vi "Server.vi"() -> ()   [LabVIEW 2021]
uses:
  <vilib>/Utility/miscctls.llb/LVPositionTypeDef.ctl
  MessageType.ctl
  <vilib>/event_ctls.llb/eventsource.ctl
panel:
  in  "stop":bool
  in  "State Change":bool=TRUE
  out "GS":enum16{"Player 1 shoot", "Player 2 Shoot"}(ring)
  out "Status":string
  out "Player 1":u8
  out "Player 2 Score":u8
  in  "Goal Post":cluster{"left":i16, "Size":i16}={"left"=110, "Size"=125}
  out "Goal Post":T1={"left"=110, "top"=0, "right"=235, "bottom"=15}
  out "Box":T1={"left"=139, "top"=147, "right"=181, "bottom"=180}
  out "goal?":bool=TRUE
  out "Del GK":dbl
  out "Defend":bool
  in  "GK":cluster{"horizontal":dbl, "vertical":dbl}={"horizontal"=175.0, "vertical"=20.0}
  in  "Box Size":cluster{"horizontal":dbl, "Vertical":dbl}={"horizontal"=21.0, "Vertical"=33.0}
  in  "Reset":bool
  out "del x":dbl=-0.26666666666666666
  in  "wait":u32=10
  in  "shot?":bool
  in  "Power":dbl(slide)=1.4141414141414141 scale=0.0..10.0
  in  "Ball Size":i16=9
  in  "Ball":cluster{"horizontal":dbl, "vertical":dbl}={"horizontal"=160.0, "vertical"=180.0}
  in  "Shoot":bool
  out "Ground":picture
  # "PLAYER 1"
  # "Misc. Controls"
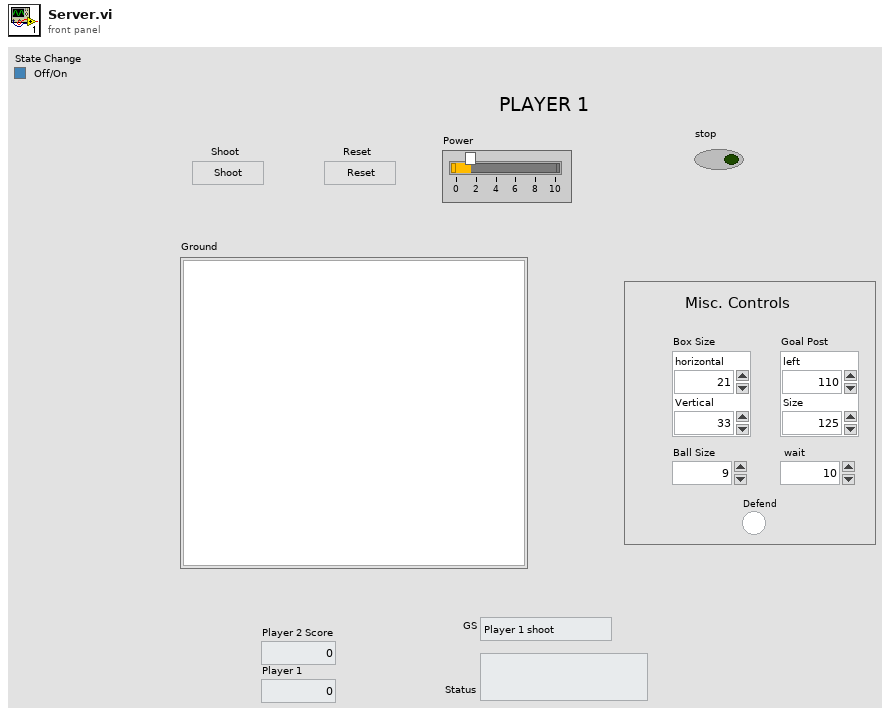
[diagram p1: front panel]
types:
  T1 = cluster{"left":i16, "top":i16, "right":i16, "bottom":i16}
  T2 = typedef "MessageType.ctl" = enum16{"Shoot", "Defend", "Reset", "Score"}
  T3 = typedef "LVPositionTypeDef.ctl" = cluster{"Left":i32, "Top":i32}
  T4 = typedef "LVPoint32TypeDef.ctl" = cluster{"Horizontal":i32, "Vertical":i32}
  T5 = typedef "eventsource.ctl" = u32
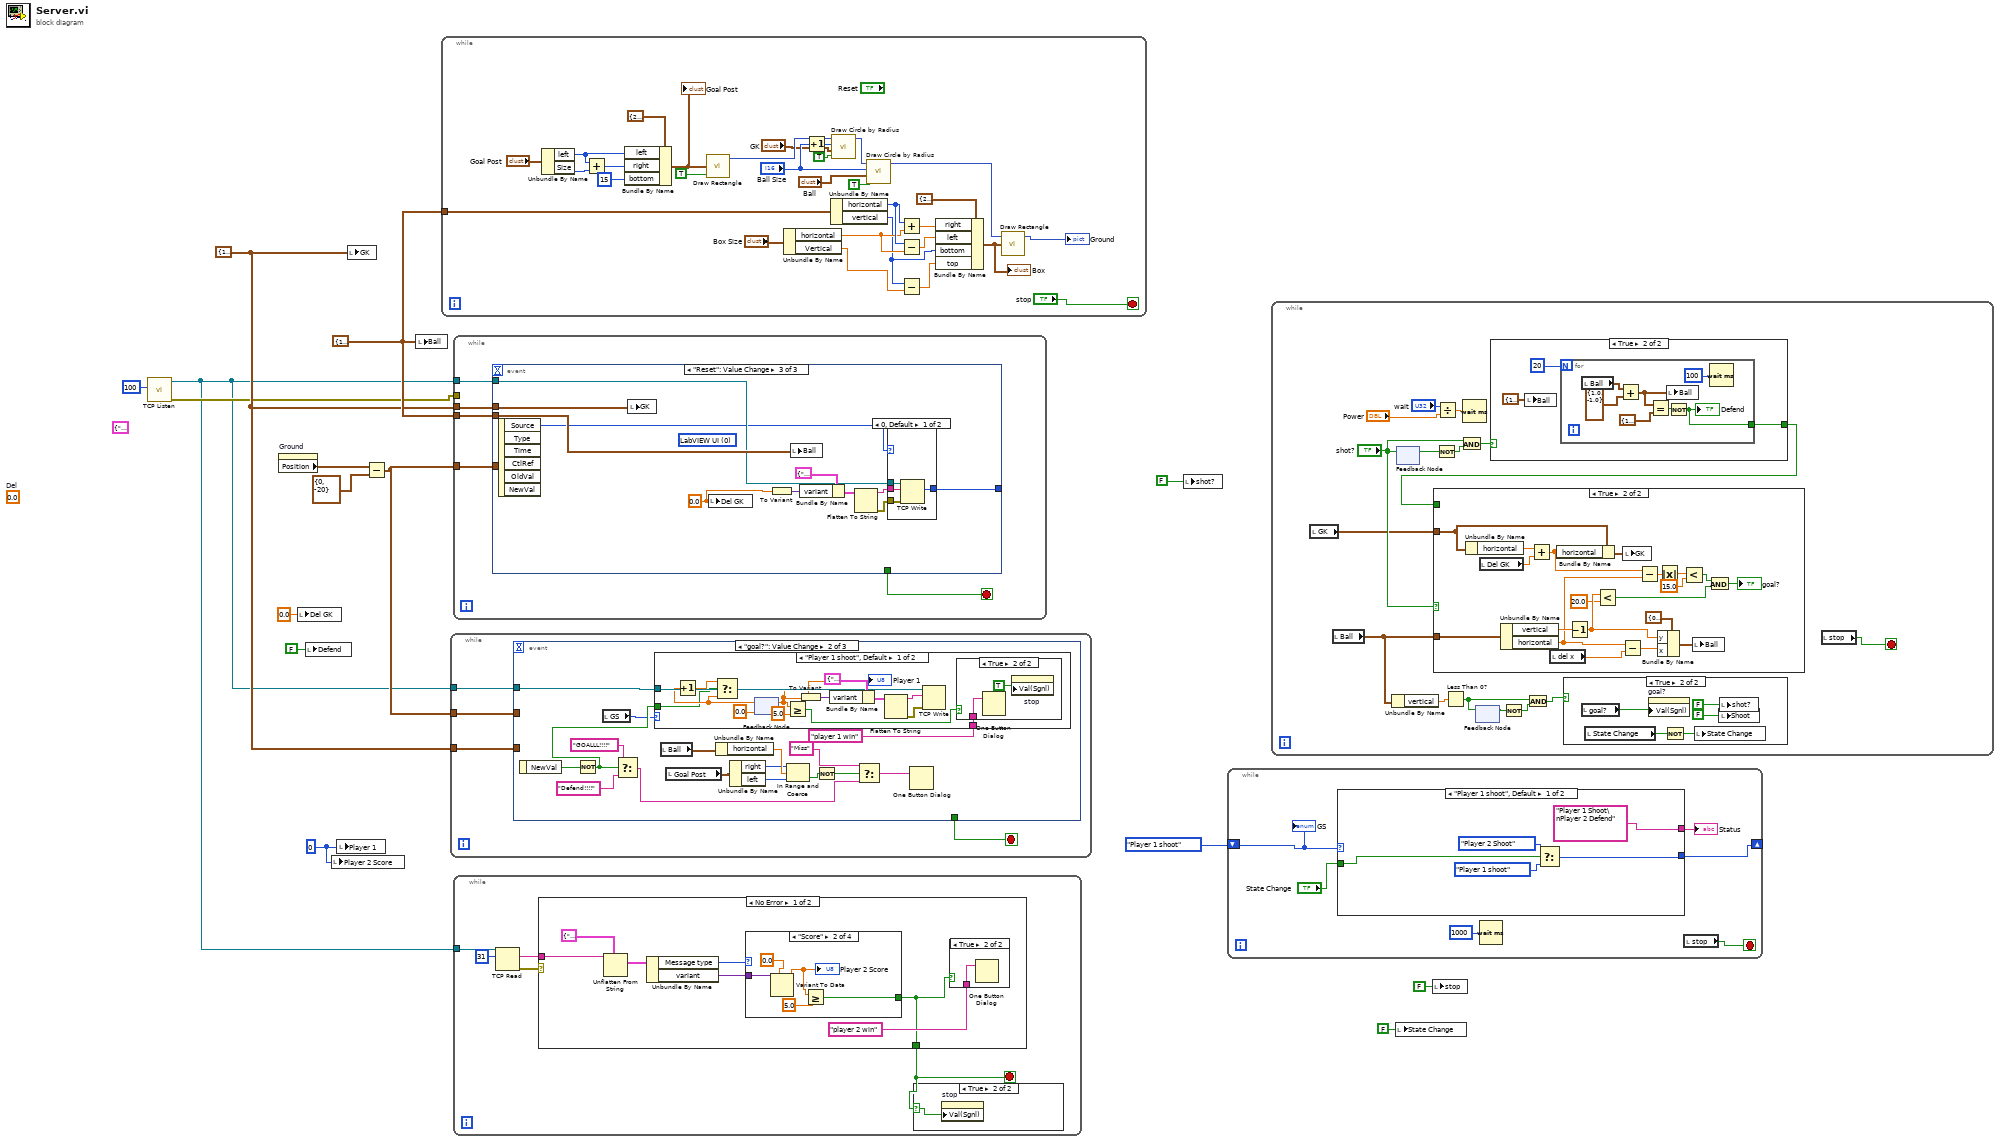
[diagram p0: block diagram]
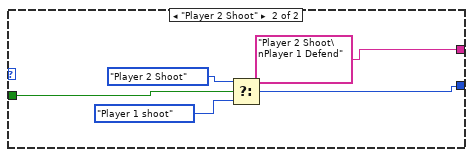
[diagram p2: hidden frame]
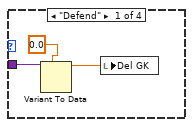
[diagram p5: hidden frame]
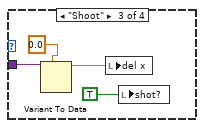
[diagram p6: hidden frame]
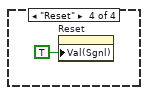
[diagram p7: hidden frame]
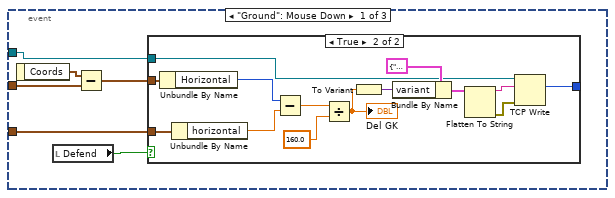
[diagram p9: hidden frame]
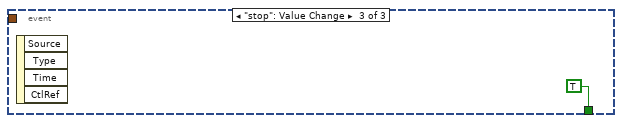
[diagram p13: hidden frame]
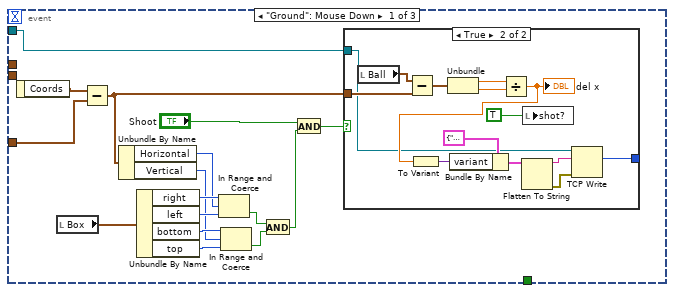
[diagram p17: hidden frame]
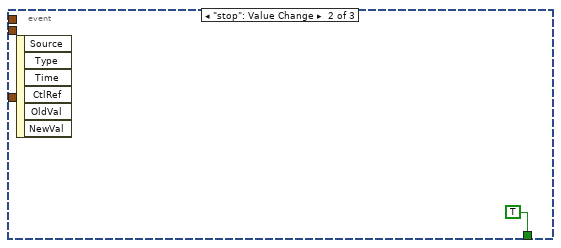
[diagram p19: hidden frame]
diagram:
  w4 = u8 0 ("Player 1")
  (unwired) 0.0  # Del
  (unwired) cluster{"Message type":T2, "variant":variant} {"Message type"=enum."Reset", "variant"=variant}
  w9 = cluster{"horizontal":dbl, "vertical":dbl} {"horizontal"=175.0, "vertical"=20.0} ("GK")
  w12 = cluster{"horizontal":i16, "vertical":i16} {"horizontal"=160, "vertical"=180} ("Ball")
  n1 = call <vilib>:"TCP Listen.vi"("port"=u16 100) -> ("error out"=w6:errorcluster, "connection ID"=w5:refnum<k5>)  [unwired: 6 in, 3 out]
  n2 = property on="Ground" class="Pict"() -> ("Position"=w14:T3)  [unwired: 2 in, 2 out]
  n3 = local write "Del GK"(0.0 ("Del GK")) -> ()
  n4 = local write "Defend"(FALSE ("def")) -> ()
  n5 = local write "Player 2 Score"(w4) -> ()
  n6 = local write "Player 1"(w4) -> ()
  n7 = local write "GK"(w9) -> ()
  n8 = Subtract(x=w14, y=T3 {"Left"=0, "Top"=-20}) -> (x-y=w11:T3)
  n9 = local write "Ball"(w12) -> ()
  n10 = while {
    tunnel: w12 -> [w26]
    stop <- "stop" stop-if-true
    n11 = Unbundle By Name("Goal Post") -> ("left"=w18:i16, "Size"=w17:i16)
    n12 = Add(x=w18, y=w17) -> (x+y=w41:i16)
    n13 = Bundle By Name(cluster=T1 {"left"=22, "top"=0, "right"=10, "bottom"=10} ("rect"), "left"=w18, "right"=w41, "bottom"=i16 15) -> (w42:T1)
    "Goal Post" <- w42
    n14 = call <vilib>:"Draw Rectangle.vi"("rect"=w42, "fill?(F)"=TRUE) -> ("new picture"=w23:picture)  [unwired: 7 in]
    n15 = Unbundle By Name("Box Size") -> ("horizontal"=w34:dbl, "Vertical"=w31:dbl)
    n16 = Increment(x="Ball Size") -> (x+1=w20:i16)
    n17 = Unbundle By Name(w26) -> ("horizontal"=w35:i16, "vertical"=w33:i16)
    n18 = call <vilib>:"Draw Circle by Radius.vi"("fill?(F)"=TRUE, "pixel center"="GK", "radius"=w20, "picture"=w23) -> ("new picture"=w21:picture)  [unwired: 7 in]
    n19 = call <vilib>:"Draw Circle by Radius.vi"("fill?(F)"=TRUE, "pixel center"="Ball", "radius"="Ball Size", "picture"=w21) -> ("new picture"=w28:picture)  [unwired: 7 in]
    n20 = Add(x=w35, y=w34) -> (x+y=w36:dbl)
    n21 = Subtract(x=w35, y=w34) -> (x-y=w32:dbl)
    n22 = Subtract(x=w33, y=w31) -> (x-y=w30:dbl)
    n23 = Bundle By Name(cluster=T1 {"left"=22, "top"=0, "right"=10, "bottom"=10} ("rect"), "right"=w36, "left"=w32, "bottom"=w33, "top"=w30) -> (w29:T1)
    "Box" <- w29
    n24 = call <vilib>:"Draw Rectangle.vi"("picture"=w28, "rect"=w29) -> ("new picture"=→"Ground":picture)  [unwired: 7 in]
  }
  n25 = while {
    tunnel: w11 -> [w49]
    tunnel: w9 -> [w48]
    tunnel: w5 -> [w47]
    stop <- w46 stop-if-true
    n26 = event shown="[1] \"goal?\": Value Change" {
      selector: _ -> [_ _ _]
      dyn-events: _ -> [_ _ _]
      timeout: _ -> [_ _ _]
      tunnel: w49 -> [w54 _ _]
      tunnel: w48 -> [w52 _ _]
      tunnel: w47 -> [w50 w73 _]
      tunnel: [_ _ TRUE] -> w46
      event "Ground": Mouse Down {
        n27 = event-data() -> ("Coords"=w55:T4)  [unwired: 1 in]
        n28 = local read "Defend"() -> (w51:bool)
        n29 = Subtract(x=w55, y=w54) -> (x-y=w53:T4)
        n30 = case shown="True" w51 {
          tunnel: w53 -> [_ w69]
          tunnel: w52 -> [_ w68]
          tunnel: w50 -> [_ w58]
          tunnel: [_ w56] -> _
          frame False {
          }
          frame True {
            n31 = Unbundle By Name(w69) -> ("Horizontal"=w67:i32)
            n32 = Unbundle By Name(w68) -> ("horizontal"=w66:dbl)
            n33 = Subtract(x=w67, y=w66) -> (x-y=w65:dbl)
            n34 = Divide(x=w65, y=160.0) -> (x/y=w57:dbl)
            "Del GK" <- w57
            n35 = To Variant(anything=w57) -> (Variant=w62:variant)
            n36 = Bundle By Name(cluster=cluster{"Message type":T2, "variant":variant} {"Message type"=enum."Defend", "variant"=variant}, "variant"=w62) -> (w61:cluster{"Message type":T2, "variant":variant})
            n37 = Flatten To String(anything=w61) -> (data string=w59:string, error out=w60:errorcluster)  [unwired: 3 in, 1 out]
            n38 = TCP Write(connection ID=w58, data in=w59, error in (no error)=w60) -> (bytes written=w56:i32)  [unwired: 1 in, 2 out]
          }
        }
      }
      event "goal?": Value Change {
        n39 = event-data() -> ("NewVal"=w86:bool)  [unwired: 1 in]
        n40 = Not(x=w86) -> (.not. x?=w72:bool)
        n41 = local read "GS"() -> (w71:enum16{"Player 1 shoot", "Player 2 Shoot"})
        n42 = Select(t="GOALLL!!!!", s=w72, f="Defend!!!!") -> (s? t:f=w75:string)
        n43 = case shown="\"Player 1 shoot\", Default" w71 {
          tunnel: w73 -> [w95 _]
          tunnel: w72 -> [w92 _]
          tunnel: "player 1 win" -> [w87 _]
          frame "Player 1 shoot", Default {
            n44 = feedback #1(0.0) -> (w93:dbl)
            n45 = Increment(x=w93) -> (x+1=w94:dbl)
            n46 = Select(t=w94, s=w92, f=w93) -> (s? t:f=w90:dbl)
            "Player 1" <- w90
            n47 = feedback-in #1(w90) -> ()
            n48 = Greater Or Equal?(x=w90, y=5.0) -> (x >= y?=w88:bool)
            n49 = To Variant(anything=w90) -> (Variant=w99:variant)
            n50 = Bundle By Name(cluster=cluster{"Message type":T2, "variant":variant} {"Message type"=enum."Score", "variant"=variant}, "variant"=w99) -> (w98:cluster{"Message type":T2, "variant":variant})
            n51 = Flatten To String(anything=w98) -> (data string=w96:string, error out=w97:errorcluster)  [unwired: 3 in, 1 out]
            n52 = TCP Write(connection ID=w95, data in=w96, error in (no error)=w97) -> ()  [unwired: 1 in, 3 out]
            n53 = case shown="True" w88 {
              tunnel: w87 -> [_ w102]
              frame False {
              }
              frame True {
                n54 = One Button Dialog(message=w102) -> ()  [unwired: 1 in, 1 out]
                n55 = property on="stop" class="Bool (strict)"("Val(Sgnl)"=TRUE ("Value (Signaling)")) -> ()  [unwired: 2 in, 2 out]
              }
            }
          }
          frame "Player 2 Shoot" {
          }
        }
        n56 = local read "Ball"() -> (w79:cluster{"horizontal":dbl, "vertical":dbl})
        n57 = local read "Goal Post"() -> (w80:T1)
        n58 = Unbundle By Name(w79) -> ("horizontal"=w83:dbl)
        n59 = Unbundle By Name(w80) -> ("right"=w81:i16, "left"=w82:i16)
        n60 = In Range and Coerce(upper limit=w81, x=w83, lower limit=w82) -> (In Range?=w78:bool)  [unwired: 1 out]
        n61 = Not(x=w78) -> (.not. x?=w74:bool)
        n62 = Select(t="Miss", s=w74, f=w75) -> (s? t:f=w76:string)
        n63 = One Button Dialog(message=w76) -> ()  [unwired: 1 in, 1 out]
      }
      event "stop": Value Change {
        n64 = event-data() -> ()  [unwired: 1 in, 4 out]
      }
    }
  }
  n65 = while {
    tunnel: w11 -> [w108]
    tunnel: w12 -> [w107]
    tunnel: w9 -> [w106]
    tunnel: w5 -> [w105]
    tunnel: w6 -> [_]
    stop <- w104 stop-if-true
    n66 = event shown="[2] \"Reset\": Value Change" {
      selector: _ -> [_ _ _]
      dyn-events: _ -> [_ _ _]
      timeout: _ -> [_ _ _]
      tunnel: w108 -> [w122 _ _]
      tunnel: w107 -> [_ _ w150]
      tunnel: w106 -> [_ _ w149]
      tunnel: w105 -> [w110 _ w143]
      tunnel: [_ _ w141] -> _
      tunnel: [_ TRUE _] -> w104
      event "Ground": Mouse Down {
        n67 = event-data() -> ("Coords"=w123:T4)  [unwired: 1 in]
        n68 = local read "Box"() -> (w121:T1)
        n69 = Subtract(x=w123, y=w122) -> (x-y=w116:T4)
        n70 = Unbundle By Name(w116) -> ("Horizontal"=w115:i32, "Vertical"=w114:i32)
        n71 = Unbundle By Name(w121) -> ("right"=w120:i16, "left"=w119:i16, "bottom"=w118:i16, "top"=w117:i16)
        n72 = In Range and Coerce(upper limit=w120, x=w115, lower limit=w119) -> (In Range?=w112:bool)  [unwired: 1 out]
        n73 = In Range and Coerce(upper limit=w118, x=w114, lower limit=w117) -> (In Range?=w113:bool)  [unwired: 1 out]
        n74 = And(x=w112, y=w113) -> (x .and. y?=w109:bool)
        n75 = And(x="Shoot", y=w109) -> (x .and. y?=w111:bool)
        n76 = case shown="True" w111 {
          tunnel: w116 -> [_ w137]
          tunnel: w110 -> [_ w126]
          tunnel: [_ w125] -> _
          frame False {
          }
          frame True {
            n77 = local read "Ball"() -> (w136:cluster{"horizontal":dbl, "vertical":dbl})
            n78 = Subtract(x=w136, y=w137) -> (x-y=w135:cluster{dbl, dbl})
            n79 = Unbundle(w135) -> (w134:dbl, w133:dbl)
            n80 = Divide(x=w134, y=w133) -> (x/y=w131:dbl)
            "del x" <- w131
            n81 = To Variant(anything=w131) -> (Variant=w130:variant)
            n82 = Bundle By Name(cluster=cluster{"Message type":T2, "variant":variant} {"Message type"=enum."Shoot", "variant"=variant}, "variant"=w130) -> (w129:cluster{"Message type":T2, "variant":variant})
            n83 = Flatten To String(anything=w129) -> (data string=w127:string, error out=w128:errorcluster)  [unwired: 3 in, 1 out]
            n84 = local write "shot?"(TRUE ("Checkbox")) -> ()
            n85 = TCP Write(connection ID=w126, data in=w127, error in (no error)=w128) -> (bytes written=w125:i32)  [unwired: 1 in, 2 out]
          }
        }
      }
      event "stop": Value Change {
        n86 = event-data() -> ()  [unwired: 1 in, 6 out]
      }
      event "Reset": Value Change {
        (unwired) T5 0 items=["LabVIEW UI"=0, "ActiveX"=1, "User Event"=25] ("Source")
        w142 = 0.0
        n87 = event-data() -> ("Source"=w140:T5)  [unwired: 1 in, 5 out]
        n88 = local write "GK"(w149) -> ()
        n89 = local write "Del GK"(w142) -> ()
        n90 = To Variant(anything=w142) -> (Variant=w147:variant)
        n91 = local write "Ball"(w150) -> ()
        n92 = Bundle By Name(cluster=cluster{"Message type":T2, "variant":variant} {"Message type"=enum."Reset", "variant"=variant}, "variant"=w147) -> (w146:cluster{"Message type":T2, "variant":variant})
        n93 = Flatten To String(anything=w146) -> (data string=w144:string, error out=w145:errorcluster)  [unwired: 3 in, 1 out]
        n94 = case shown="0, Default" w140 {
          tunnel: w145 -> [w154 _]
          tunnel: w144 -> [w153 _]
          tunnel: w143 -> [w152 _]
          tunnel: [w151 _] -> w141
          frame 0, Default {
            n95 = TCP Write(connection ID=w152, data in=w153, error in (no error)=w154) -> (bytes written=w151:i32)  [unwired: 1 in, 2 out]
          }
          frame 1 {
          }
        }
      }
    }
  }
  n96 = while {
    tunnel: w5 -> [w159]
    stop <- w155 stop-if-true
    n97 = TCP Read(connection ID=w159, bytes to read=31) -> (data out=w156:string, error out=w157:errorcluster)  [unwired: 3 in, 1 out]
    n98 = case shown="No Error" w157 {
      tunnel: w156 -> [w167 _]
      tunnel: [w161 _] -> w155
      frame No Error {
        n99 = Unflatten From String(type=cluster{"Message type":T2, "variant":variant} {"Message type"=enum."Defend", "variant"=variant}, binary string=w167) -> (value=w165:cluster{"Message type":T2, "variant":variant})  [unwired: 3 in, 2 out]
        n100 = Unbundle By Name(w165) -> ("Message type"=w164:T2, "variant"=w163:variant)
        n101 = case shown="\"Score\"" w164 {
          tunnel: w163 -> [w171 w176 w180 _]
          tunnel: [_ w172 _ _] -> w161
          frame "Defend" {
            n102 = Variant To Data(type=0.0 ("x/y"), Variant=w171) -> (data=w169:dbl)  [unwired: 1 in, 1 out]
            n103 = local write "Del GK"(w169) -> ()
          }
          frame "Score" {
            n104 = Variant To Data(type=0.0 ("x/y"), Variant=w176) -> (data=w174:dbl)  [unwired: 1 in, 1 out]
            "Player 2 Score" <- w174
            n105 = Greater Or Equal?(x=w174, y=5.0) -> (x >= y?=w172:bool)
          }
          frame "Shoot" {
            n106 = Variant To Data(type=0.0 ("x/y"), Variant=w180) -> (data=w178:dbl)  [unwired: 1 in, 1 out]
            n107 = local write "del x"(w178) -> ()
            n108 = local write "shot?"(TRUE ("Checkbox")) -> ()
          }
          frame "Reset" {
            n109 = property on="Reset" class="Bool (strict)"("Val(Sgnl)"=TRUE ("Value (Signaling)")) -> ()  [unwired: 2 in, 2 out]
          }
        }
        n110 = case shown="True" w161 {
          tunnel: "player 2 win" -> [_ w168]
          frame False {
          }
          frame True {
            n111 = One Button Dialog(message=w168) -> ()  [unwired: 1 in, 1 out]
          }
        }
      }
      frame Error {
      }
    }
    n112 = case shown="True" w155 {
      selector: w155 -> [_ w160]
      frame False {
      }
      frame True {
        n113 = property on="stop" class="Bool (strict)"("Val(Sgnl)"=w160) -> ()  [unwired: 2 in, 2 out]
      }
    }
  }
  n114 = local write "shot?"(FALSE ("Checkbox")) -> ()
  n115 = while {
    shift-right: [w184] -> _
    shift-left: enum16{"Player 1 shoot", "Player 2 Shoot"}."Player 1 shoot" -> [w187]
    stop <- w182 stop-if-true
    n116 = case shown="\"Player 1 shoot\", Default" w187 {
      tunnel: ["Player 1 Shoot\nPlayer 2 Defend" "Player 2 Shoot\nPlayer 1 Defend"] -> w186
      tunnel: [w189 w194] -> w184
      tunnel: "State Change" -> [w188 w193]
      frame "Player 1 shoot", Default {
        n117 = Select(t=enum16{"Player 1 shoot", "Player 2 Shoot"}."Player 2 Shoot", s=w188, f=enum16{"Player 1 shoot", "Player 2 Shoot"}."Player 1 shoot") -> (s? t:f=w189:enum16{"Player 1 shoot", "Player 2 Shoot"})
      }
      frame "Player 2 Shoot" {
        n118 = Select(t=enum16{"Player 1 shoot", "Player 2 Shoot"}."Player 2 Shoot", s=w193, f=enum16{"Player 1 shoot", "Player 2 Shoot"}."Player 1 shoot") -> (s? t:f=w194:enum16{"Player 1 shoot", "Player 2 Shoot"})
      }
    }
    "Status" <- w186
    n119 = Wait (ms)(milliseconds to wait=u32 1000) -> ()  [unwired: 1 out]
    n120 = local read "stop"() -> (w182:bool)
    "GS" <- w187
  }
  n121 = while {
    stop <- w198 stop-if-true
    n122 = local read "GK"() -> (w204:cluster{"horizontal":dbl, "vertical":dbl})
    n123 = local read "Ball"() -> (w210:cluster{"horizontal":dbl, "vertical":dbl})
    n124 = Unbundle By Name(w210) -> ("vertical"=w209:dbl)
    n125 = feedback-in #2("shot?") -> ()
    n126 = feedback #2() -> (w208:bool)  [unwired: 1 in]
    n127 = Not(x=w208) -> (.not. x?=w206:bool)
    n128 = Divide(x="wait", y="Power") -> (x/y=w212:dbl)
    n129 = Less Than 0?(x=w209) -> (x < 0?=w203:bool)
    n130 = And(x="shot?", y=w206) -> (x .and. y?=w205:bool)
    n131 = Wait (ms)(milliseconds to wait=w212) -> ()  [unwired: 1 out]
    n132 = feedback #3() -> (w201:bool)  [unwired: 1 in]
    n133 = feedback-in #3(w203) -> ()
    n134 = case shown="True" w205 {
      tunnel: [_ w214] -> w199
      frame False {
      }
      frame True {
        n135 = local write "Ball"(cluster{"horizontal":i16, "vertical":i16} {"horizontal"=140, "vertical"=200} ("Ball")) -> ()
        n136 = for {
          N: 20 -> [_]
          tunnel: [w217] -> w214
          n137 = local read "Ball"() -> (w223:cluster{"horizontal":dbl, "vertical":dbl})
          n138 = Add(x=w223, y=cluster{"horizontal":dbl, "vertical":dbl} {"horizontal"=1.0, "vertical"=-1.0}) -> (x+y=w220:cluster{"horizontal":dbl, "vertical":dbl})
          n139 = Equal?(x=w220, y=cluster{"horizontal":i16, "vertical":i16} {"horizontal"=160, "vertical"=180} ("Ball")) -> (x = y?=w219:bool)
          n140 = local write "Ball"(w220) -> ()
          n141 = Not(x=w219) -> (.not. x?=w217:bool)
          "Defend" <- w217
          n142 = Wait (ms)(milliseconds to wait=u32 100) -> ()  [unwired: 1 out]
        }
      }
    }
    n143 = case shown="True" "shot?" {
      tunnel: w210 -> [_ w243]
      tunnel: w204 -> [_ w242]
      tunnel: w199 -> [_ _]
      frame False {
      }
      frame True {
        n144 = Unbundle By Name(w242) -> ("horizontal"=w241:dbl)
        n145 = local read "Del GK"() -> (w240:dbl)
        n146 = Unbundle By Name(w243) -> ("vertical"=w247:dbl, "horizontal"=w235:dbl)
        n147 = Add(x=w241, y=w240) -> (x+y=w236:dbl)
        n148 = local read "del x"() -> (w248:dbl)
        n149 = Bundle By Name(cluster=w242, "horizontal"=w236) -> (w239:cluster{"horizontal":dbl, "vertical":dbl})
        n150 = Decrement(x=w247) -> (x-1=w238:dbl)
        n151 = Less?(x=w238, y=20.0) -> (x < y?=w230:bool)
        n152 = Subtract(x=w235, y=w248) -> (x-y=w245:dbl)
        n153 = local write "GK"(w239) -> ()
        n154 = Subtract(x=w236, y=w235) -> (x-y=w234:dbl)
        n155 = Bundle By Name(cluster=cluster{"x":dbl, "y":dbl} {"x"=0.0, "y"=0.0}, "y"=w238, "x"=w245) -> (w244:cluster{"x":dbl, "y":dbl})
        n156 = Absolute Value(x=w234) -> (abs(x)=w233:dbl)
        n157 = Less?(x=w233, y=15.0) -> (x < y?=w231:bool)
        n158 = local write "Ball"(w244) -> ()
        n159 = And(x=w231, y=w230) -> (x .and. y?=→"goal?":bool)
      }
    }
    n160 = Not(x=w201) -> (.not. x?=w200:bool)
    n161 = And(x=w203, y=w200) -> (x .and. y?=w202:bool)
    n162 = case shown="True" w202 {
      frame False {
      }
      frame True {
        n163 = local read "goal?"() -> (w226:bool)
        n164 = local read "State Change"() -> (w225:bool)
        n165 = property on="goal?" class="Bool (strict)"("Val(Sgnl)"=w226) -> ()  [unwired: 2 in, 2 out]
        n166 = Not(x=w225) -> (.not. x?=w224:bool)
        n167 = local write "State Change"(w224) -> ()
        n168 = local write "Shoot"(FALSE ("Checkbox")) -> ()
        n169 = local write "shot?"(FALSE ("Checkbox")) -> ()
      }
    }
    n170 = local read "stop"() -> (w198:bool)
  }
  n171 = local write "State Change"(FALSE ("State Change")) -> ()
  n172 = local write "stop"(FALSE ("stop")) -> ()
